vi "TestExecution.vi"(8 "error in (no error)":errorcluster, 11 "TestRunner in":refnum<class "TestRunner.lvclass">) -> (0 "error out":errorcluster, 3 "TestRunner out":refnum<class "TestRunner.lvclass">)   [LabVIEW 2019, in "TestRunner.lvlib" / "TestRunner.lvclass"]
uses:
  TestRunner.lvclass
  C:/Program Files (x86)/National Instruments/LabVIEW 2019/vi.lib/NI/Event Source Actor/Event Source/Event Source/Event Source.lvclass
  TestRunnerEvent.lvclass
  C:/Program Files (x86)/National Instruments/LabVIEW 2019/vi.lib/NI/Event Source Actor/Event Source/Event/Event.lvclass
  <vilib>/NI/Event Source Actor/Event Source/Event/Event.lvclass/Event.ctl
  <vilib>/NI/Event Source Actor/Event Source/Event/Event.lvclass
  <vilib>/NI/Event Source Actor/Event Source/Event Source/Event Source.lvclass
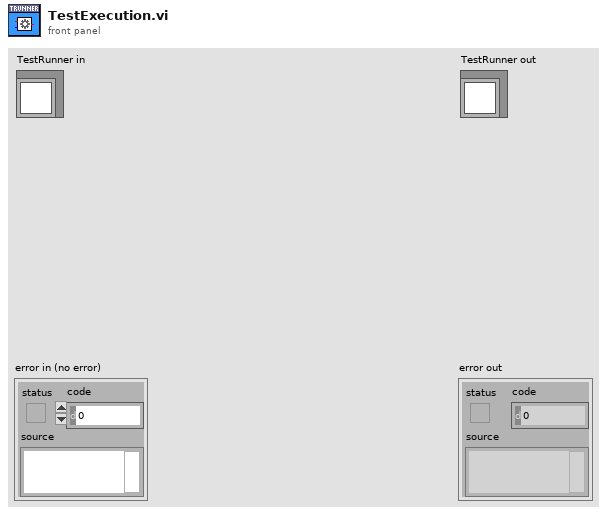
[diagram p1: front panel]
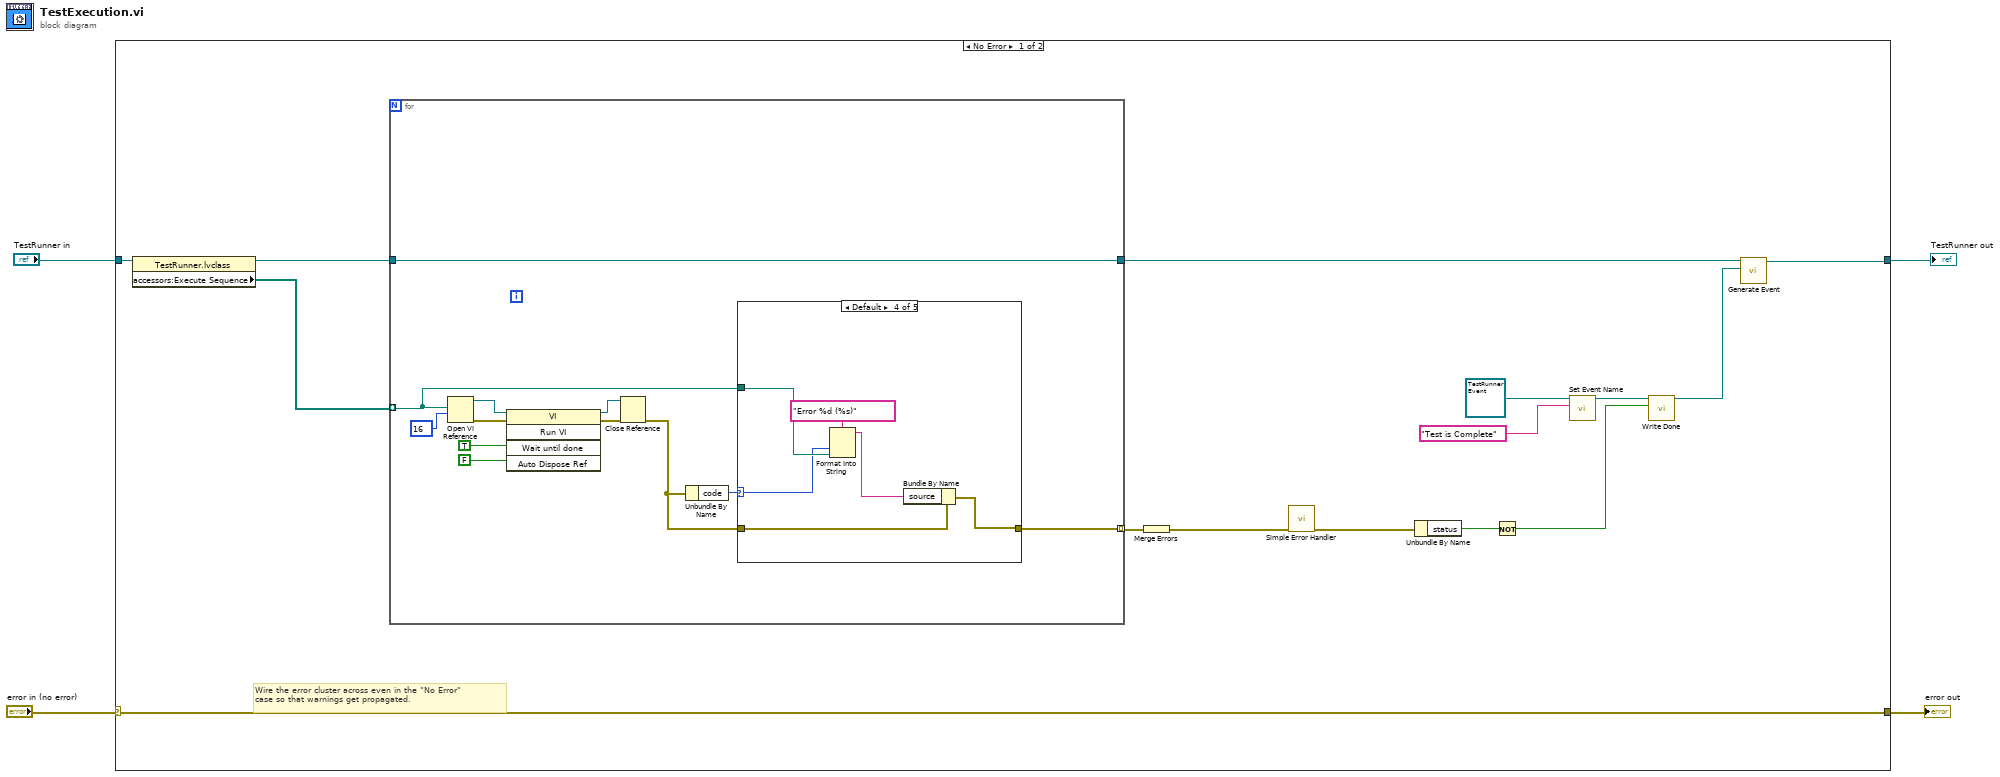
[diagram p0: block diagram]
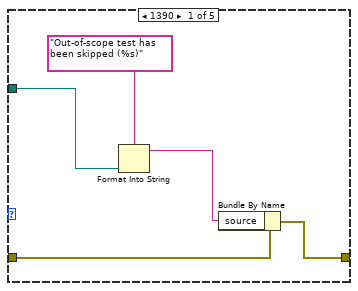
[diagram p2: hidden frame]
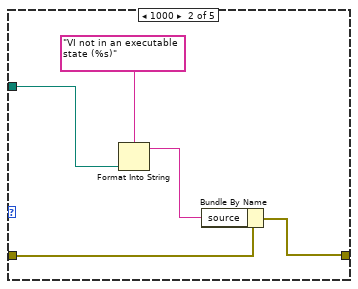
[diagram p3: hidden frame]
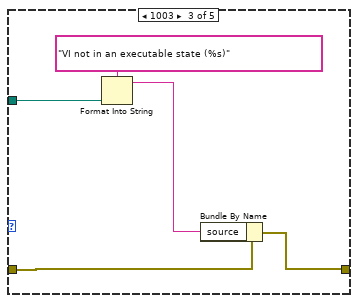
[diagram p4: hidden frame]
diagram:
  n1 = case shown="No Error" "error in (no error)" {
    selector: "error in (no error)" -> [w10 w55]
    tunnel: [w10 w55] -> w3
    tunnel: [w15 w54] -> w1
    tunnel: "TestRunner in" -> [w19 w54]
    frame No Error {
      # "Wire the error cluster across even in the \"No Error\"\ncase so that warnings get propagated."
      n2 = property class="TestRunner.lvclass"(reference=w19) -> (reference out=w6:refnum<class "TestRunner.lvclass">, "accessors:Execute Sequence"=w18:path[])  [unwired: 1 in, 1 out]
      n3 = for {
        tunnel: w18 -> [w22] mode=indexing
        tunnel: [w23] -> w9 mode=indexing
        tunnel: w6 -> [w20]
        tunnel: [w20] -> w5
        n4 = Open VI Reference(vi path=w22, options=16) -> (vi reference=w26:refnum<vi>, error out=w31:errorcluster)  [unwired: 4 in]
        n5 = invoke on="Invoke Node" class="VI" method="Run VI"(reference=w26, error in=w31, "Wait until done"=TRUE ("Wait Until Done"), "Auto Dispose Ref"=FALSE ("Auto Dispose Reference")) -> (reference out=w28:refnum<vi>, error out=w27:errorcluster)  [unwired: 1 in, 3 out]
        n6 = Close Reference(reference=w28, error in (no error)=w27) -> (error out=w24:errorcluster)
        n7 = Unbundle By Name(w24) -> ("code"=w25:i32)
        n8 = case shown="Default" w25 {
          selector: w25 -> [_ _ _ w50 _]
          tunnel: w24 -> [w34 w38 w43 w49 w53]
          tunnel: [w33 w37 w42 w47 w53] -> w23
          tunnel: w22 -> [w36 w41 w46 w52 _]
          frame 1390 {
            n9 = Format Into String(format string="Out-of-scope test has been skipped (%s)" ("Label"), w36) -> (resulting string=w32:string)  [unwired: 2 in, 1 out]
            n10 = Bundle By Name(cluster=w34, "source"=w32) -> (w33:errorcluster)
          }
          frame 1000 {
            n11 = Format Into String(format string="VI not in an executable state (%s)" ("Label"), w41) -> (resulting string=w39:string)  [unwired: 2 in, 1 out]
            n12 = Bundle By Name(cluster=w38, "source"=w39) -> (w37:errorcluster)
          }
          frame 1003 {
            n13 = Format Into String(format string="VI not in an executable state (%s)" ("Label"), w46) -> (resulting string=w44:string)  [unwired: 2 in, 1 out]
            n14 = Bundle By Name(cluster=w43, "source"=w44) -> (w42:errorcluster)
          }
          frame Default {
            n15 = Format Into String(format string="Error %d (%s)" ("Label"), w50, w52) -> (resulting string=w48:string)  [unwired: 2 in, 1 out]
            n16 = Bundle By Name(cluster=w49, "source"=w48) -> (w47:errorcluster)
          }
          frame 0 {
          }
        }
      }
      n17 = Merge Errors(w9) -> (w8:errorcluster)
      n18 = call <vilib>:"Simple Error Handler.vi"("error in (no error)"=w8) -> ("error out"=w7:errorcluster)  [unwired: 4 in, 4 out]
      n19 = Unbundle By Name(w7) -> ("status"=w12:bool)
      n20 = Not(x=w12) -> (.not. x?=w11:bool)
      n21 = call <vilib>:"Set Event Name.vi"("Name (Generic)"="Test is Complete", "Event In"=refnum<class "TestRunnerEvent.lvclass"> refnum ("UnitTestEngine.lvlib:TestRunnerEvent.lvclass")) -> ("Event Out"=w14:refnum<class "TestRunnerEvent.lvclass">)  [unwired: 9 in]
      n22 = call-dynamic "Write Done.vi"("Done"=w11, "TestRunnerEvent in"=w14) -> ("TestRunnerEvent out"=w13:refnum<class "TestRunnerEvent.lvclass">)  [unwired: 8 in, 1 out]
      n23 = call <vilib>:"Generate Event.vi"("Event"=w13, "Event Source In"=w5) -> ("Event Source Out"=w15:refnum<class "TestRunner.lvclass">)  [unwired: 8 in, 1 out]
    }
    frame Error {
    }
  }
  "error out" <- w3
  "TestRunner out" <- w1
